vi "AutonGlobals.vi"() -> ()   [LabVIEW 2017]
panel:
  out "Intake":dbl
  out "Shooter Angle":bool
  out "Shooter Pneumatic":bool
  out "Gyro Angle":dbl
  out "Shooter Power":dbl
  out "Drive Distance":dbl
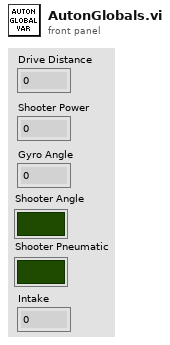
[diagram p1: front panel]
diagram:
